vi "RDS Serial Write Config.vi"(7 "Termination Char(s)":string, 8 "error in (no error)":errorcluster, 9 "baud rate":u32, 10 "VISA resource name":refnum<visa-resource-name>, 11 "RDS Serial Instrument Actor in":refnum<class "RDS Serial Instrument Actor.lvclass">) -> (0 "error out":errorcluster, 3 "RDS Serial Instrument Actor out":refnum<class "RDS Serial Instrument Actor.lvclass">)   [LabVIEW 2015, in "RDS Abstracts.lvlib" / "RDS Serial Instrument Actor.lvlib" / "RDS Serial Instrument Actor.lvclass"]
uses:
  RDS Serial Instrument Actor.lvclass
  RDS Serial Instrument Actor.lvclass/RDS Serial Instrument Actor.ctl
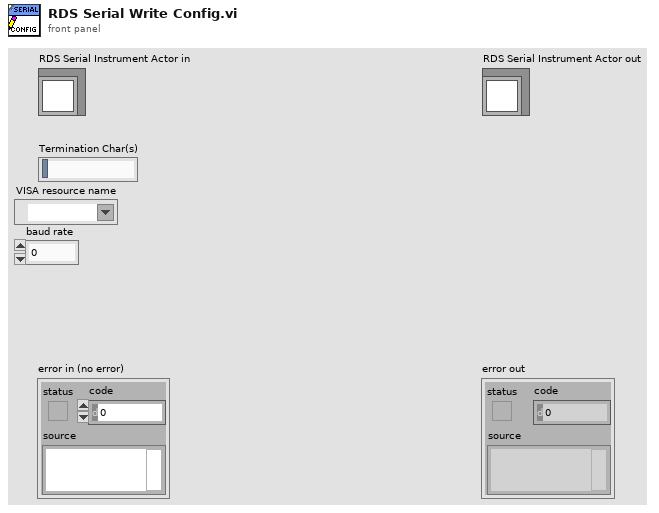
[diagram p1: front panel]
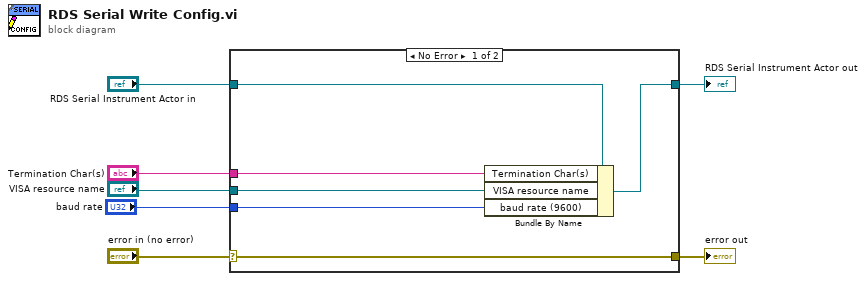
[diagram p0: block diagram]
diagram:
  n1 = case shown="No Error" "error in (no error)" {
    selector: "error in (no error)" -> [w13 w14]
    tunnel: [w13 w14] -> w6
    tunnel: [w11 w15] -> w4
    tunnel: "RDS Serial Instrument Actor in" -> [w12 w15]
    tunnel: "Termination Char(s)" -> [w10 _]
    tunnel: "VISA resource name" -> [w9 _]
    tunnel: "baud rate" -> [w8 _]
    frame No Error {
      n2 = Bundle By Name(cluster=w12, "Termination Char(s)"=w10, "VISA resource name"=w9, "baud rate (9600)"=w8) -> (w11:refnum<class "RDS Serial Instrument Actor.lvclass">)
    }
    frame Error {
    }
  }
  "error out" <- w6
  "RDS Serial Instrument Actor out" <- w4
